vi "testConfigureSystemDefinitionFile.vi"(8 "error in (no error)":errorcluster, 11 "TestCase in":refnum<class "VeriStandTestUtilitiesTests.lvclass">) -> (0 "error out":errorcluster, 3 "TestCase out":refnum<class "VeriStandTestUtilitiesTests.lvclass">)   [LabVIEW 2017, in "VeriStandTestUtilitiesTests.lvclass"]
uses:
  VeriStandTestUtilitiesTests.lvclass
  <vilib>/addons/_JKI Toolkits/VI Tester/TestCase.llb/TestCase.lvclass
  VeriStandTestUtilities.lvlib
  C:/Program Files (x86)/National Instruments/LabVIEW 2017/vi.lib/addons/_JKI Toolkits/VI Tester/TestCase.llb/TestCase.lvclass
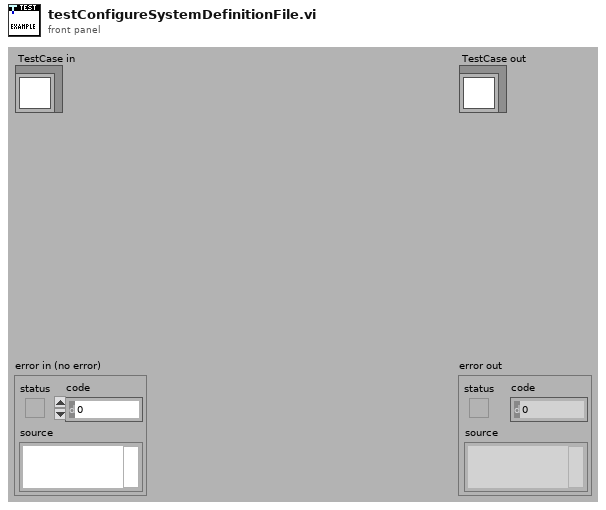
[diagram p1: front panel]
types:
  T1 = typedef "VeriStandTestUtilities.lvlib/SystemDefinitionInformation.ctl" = cluster{"Path":path, "Target Information List":T2[]}
  T2 = typedef "VeriStandTestUtilities.lvlib/TargetInformation.ctl" = cluster{"Name":string, "IP Address":string, "Operating System":string, "Target Rate":dbl, "Chassis List":T3[], "Custom Device List":string[]}
  T3 = typedef "VeriStandTestUtilities.lvlib/ChassisInformation.ctl" = cluster{"Name":string, "Devices":string[]}
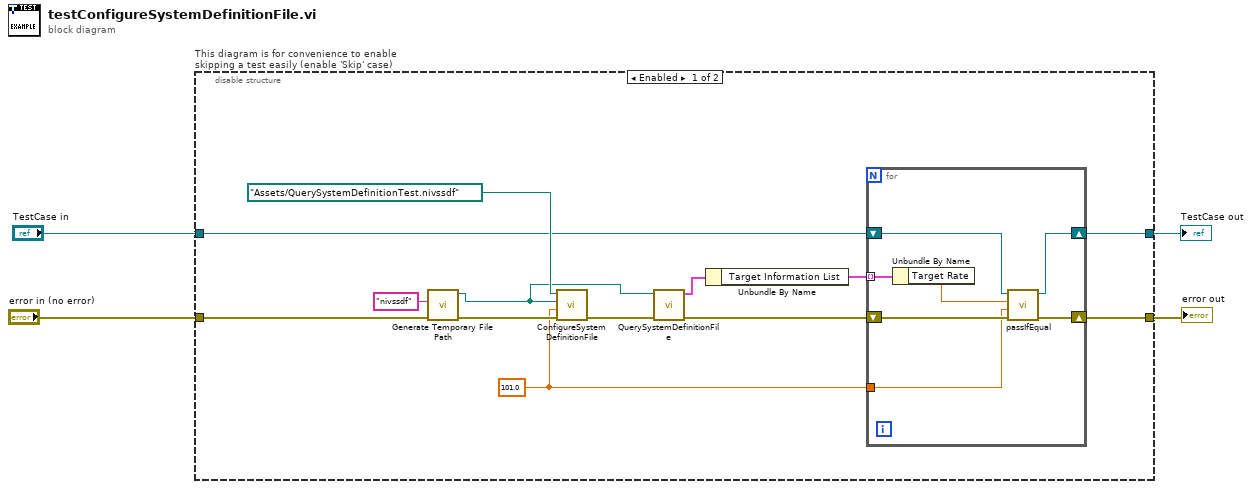
[diagram p0: block diagram]
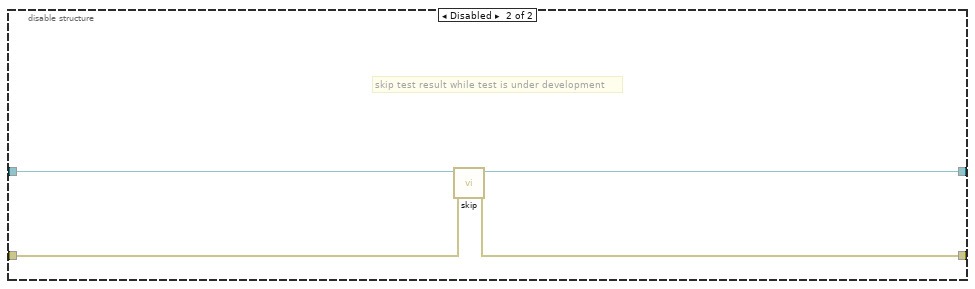
[diagram p2: hidden frame]
diagram:
  n1 = disable-structure "This diagram is for convenience to enable skipping a test easily (enable 'Skip' case)" shown="Enabled" {
    disable-tunnel: "TestCase in" -> [w9 w28]
    disable-tunnel: [w7 w26] -> w1
    disable-tunnel: [w5 w27] -> w3
    disable-tunnel: "error in (no error)" -> [w17 w25]
    frame Enabled {
      w6 = 101.0 ("Target Rate")
      n2 = call <vilib>:"Generate Temporary File Path.vi"("error in (no error)"=w17, "Temporary File Extension (tmp)"="nivssdf") -> ("error out"=w14:errorcluster, "Unique Temporary File Path"=w12:path)  [unwired: 8 in]
      n3 = call "ConfigureSystemDefinitionFile.vi"("error in (no error)"=w14, "Target Rate"=w6, "Destination System Definition File in"=w12, "Source System Definition File in"=path "Assets/QuerySystemDefinitionTest.nivssdf" ("custom device xml path")) -> ("error out"=w16:errorcluster)  [unwired: 7 in]
      n4 = call "QuerySystemDefinitionFile.vi"("error in (no error)"=w16, "System Definiton File in"=w12) -> ("error out"=w8:errorcluster, "System Definition Information out"=w11:T1)  [unwired: 8 in]
      n5 = Unbundle By Name(w11) -> ("Target Information List"=w10:T2[])
      n6 = for {
        tunnel: w10 -> [w24] mode=indexing
        shift-right: [w20] -> w7
        shift-left: w9 -> [w23]
        shift-right: [w19] -> w5
        shift-left: w8 -> [w22]
        tunnel: w6 -> [w18]
        n7 = Unbundle By Name(w24) -> ("Target Rate"=w21:dbl)
        n8 = call-dynamic "passIfEqual.vi"("error in (no error)"=w22, "y"=w18, "x"=w21, "TestCase in"=w23) -> ("error out"=w19:errorcluster, "TestCase out"=w20:refnum<class "VeriStandTestUtilitiesTests.lvclass">)  [unwired: 6 in]
      }
    }
    frame Disabled {
      # "skip test result while test is under development"
      n9 = call <vilib>:"skip.vi"("error in (no error)"=w25, "TestCase in"=w28) -> ("error out"=w27:errorcluster, "TestCase out"=w26:refnum<class "VeriStandTestUtilitiesTests.lvclass">)  [unwired: 8 in]
    }
  }
  "error out" <- w3
  "TestCase out" <- w1
